vi "core_code_plus_minus_eco.vi"(2 "code in":i32) -> (7 "code w/ ECO":i32, 9 "code w/out ECO":i32)   [LabVIEW 2015]
uses:
  polys/poly_global_eco_plus.vi
  polys/poly_global_eco_minus.vi
  core_global_ECO.vi
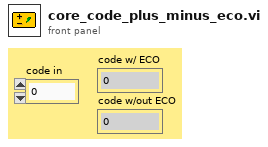
[diagram p1: front panel]
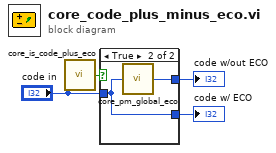
[diagram p0: block diagram]
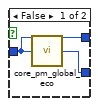
[diagram p2: hidden frame]
diagram:
  n1 = call "core_is_code_plus_eco.vi"("code"="code in") -> ("has + ECO?"=w4:bool)  [unwired: 4 in]
  n2 = case shown="True" w4 {
    tunnel: "code in" -> [w6 w8]
    tunnel: [w5 w8] -> w2
    tunnel: [w6 w7] -> w1
    frame False {
      n3 = call-poly "core_pm_global_eco.vi"("code (w/out ECO)"=w6) -> ("code (+ ECO)"=w5:i32)  [unwired: 4 in]
    }
    frame True {
      n4 = call-poly "core_pm_global_eco.vi"("code (w/ ECO)"=w8) -> ("code (- ECO)"=w7:i32)  [unwired: 4 in]
    }
  }
  "code w/ ECO" <- w2
  "code w/out ECO" <- w1
